vi "Ex3_Cluster.vi"() -> ()   [LabVIEW 2024]
panel:
  out "Device Name 2":string
  out "Device Name":string
  out "Samples":dbl[](array[numeric])
  out "Sample Rate":dbl
  in  "Signal":T1
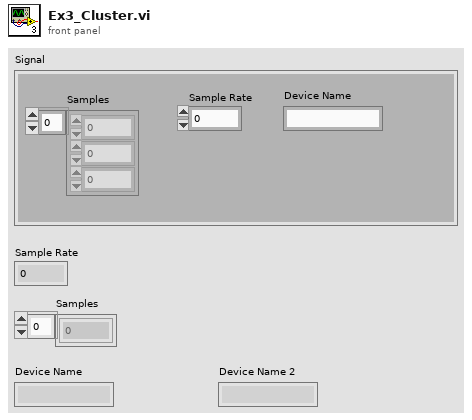
[diagram p1: front panel]
types:
  T1 = cluster{"Samples":dbl[], "Sample Rate":dbl, "Device Name":string}
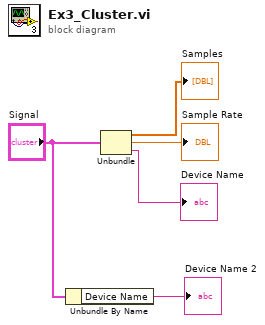
[diagram p0: block diagram]
diagram:
  n1 = Unbundle By Name("Signal") -> ("Device Name"=→"Device Name 2":string)
  n2 = Unbundle("Signal") -> ("Samples"=→"Samples":dbl[], "Sample Rate"=→"Sample Rate":dbl, "Device Name"=→"Device Name":string)
